vi "Rotate.vi"(10 "Inverse":dbl[][](array[numeric]), 11 "Inverse":bool caption="Scan") -> (2 "Array out":dbl[][](array[numeric]))   [LabVIEW 2012]
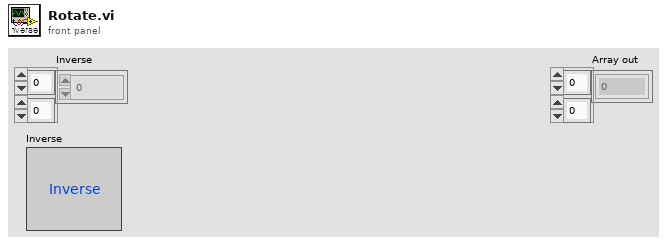
[diagram p1: front panel]
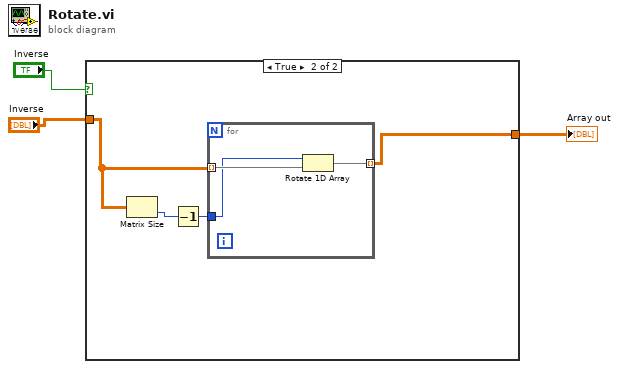
[diagram p0: block diagram]
diagram:
  n1 = case shown="True" "Inverse" {
    tunnel: "Inverse" -> [w4 w7]
    tunnel: [w4 w8] -> w1
    frame False {
    }
    frame True {
      n2 = Matrix Size(0:w7) -> (2:w6:i32)  [unwired: 1 out]
      n3 = Decrement(x=w6) -> (x-1=w5:i32)
      n4 = for {
        tunnel: w7 -> [w11] mode=indexing
        tunnel: [w10] -> w8 mode=indexing
        tunnel: w5 -> [w9]
        n5 = Rotate 1D Array(1:w11, 2:w9) -> (0:w10:dbl[])
      }
    }
  }
  "Array out" <- w1
